vi "Panel Resized.vi"(6 "Sizing Refnums":T2, 8 "error in (no error)":errorcluster, 9 "Origin":cluster{"H":i16, "V":i16}, 10 "NewBnds":T1, 11 "Size Constraints":cluster{"min tab width":i32, "w/h":dbl}) -> (0 "error out":errorcluster)   [LabVIEW 2019]
uses:
  <vilib>/Utility/miscctls.llb/LVRectTypeDef.ctl
  <vilib>/Utility/miscctls.llb/LVRowAndColumnTypeDef.ctl
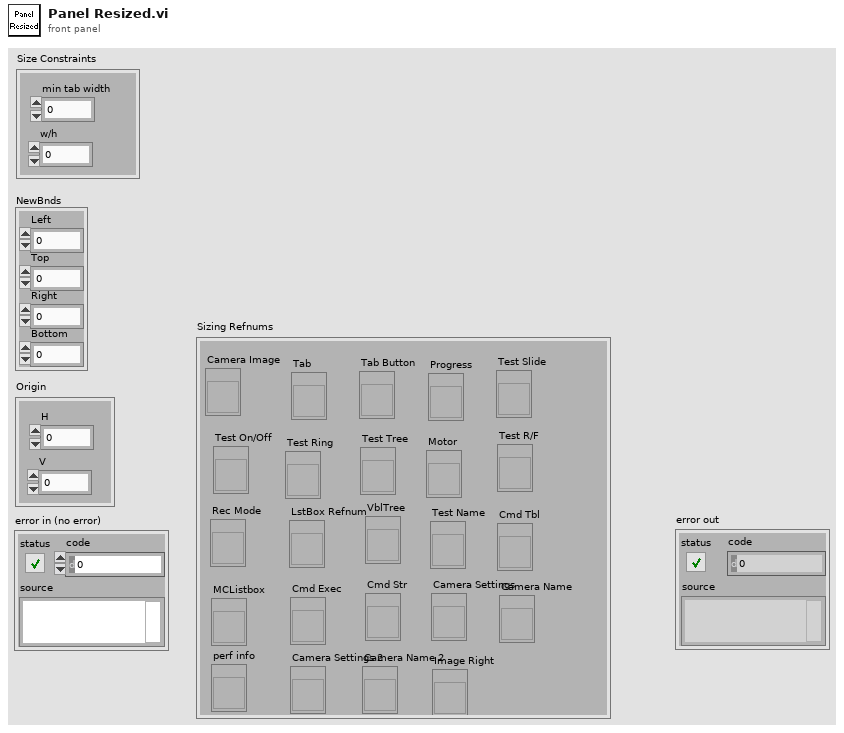
[diagram p1: front panel]
types:
  T1 = typedef "LVRectTypeDef.ctl" = cluster{"Left":i16, "Top":i16, "Right":i16, "Bottom":i16}
  T2 = cluster{"Camera Image":refnum<vi>, "Tab":refnum<vi>, "Tab Button":refnum<vi>, "Rec Mode":refnum<vi>, "Test Slide":refnum<vi>, "Test On/Off":refnum<vi>, "Test Ring":refnum<vi>, "Test R/F":refnum<vi>, "Test Name":refnum<vi>, "Motor":refnum<vi>, "Progress":refnum<vi>, "LstBox Refnum":refnum<vi>, "Test Tree":refnum<vi>, "VblTree":refnum<vi>, "Cmd Tbl":refnum<vi>, "MCListbox":refnum<vi>, "Cmd Exec":refnum<vi>, "Cmd Str":refnum<vi>, "Camera Settings":refnum<vi>, "Camera Name":refnum<vi>, "perf info":refnum<vi>, "Camera Settings 2":refnum<vi>, "Camera Name 2":refnum<vi>, "Image Right":refnum<vi>}
  T3 = typedef "LVRowAndColumnTypeDef.ctl" = cluster{"Row":i32, "Column":i32}
  T4 = typedef "LVPositionTypeDef.ctl" = cluster{"Left":i32, "Top":i32}
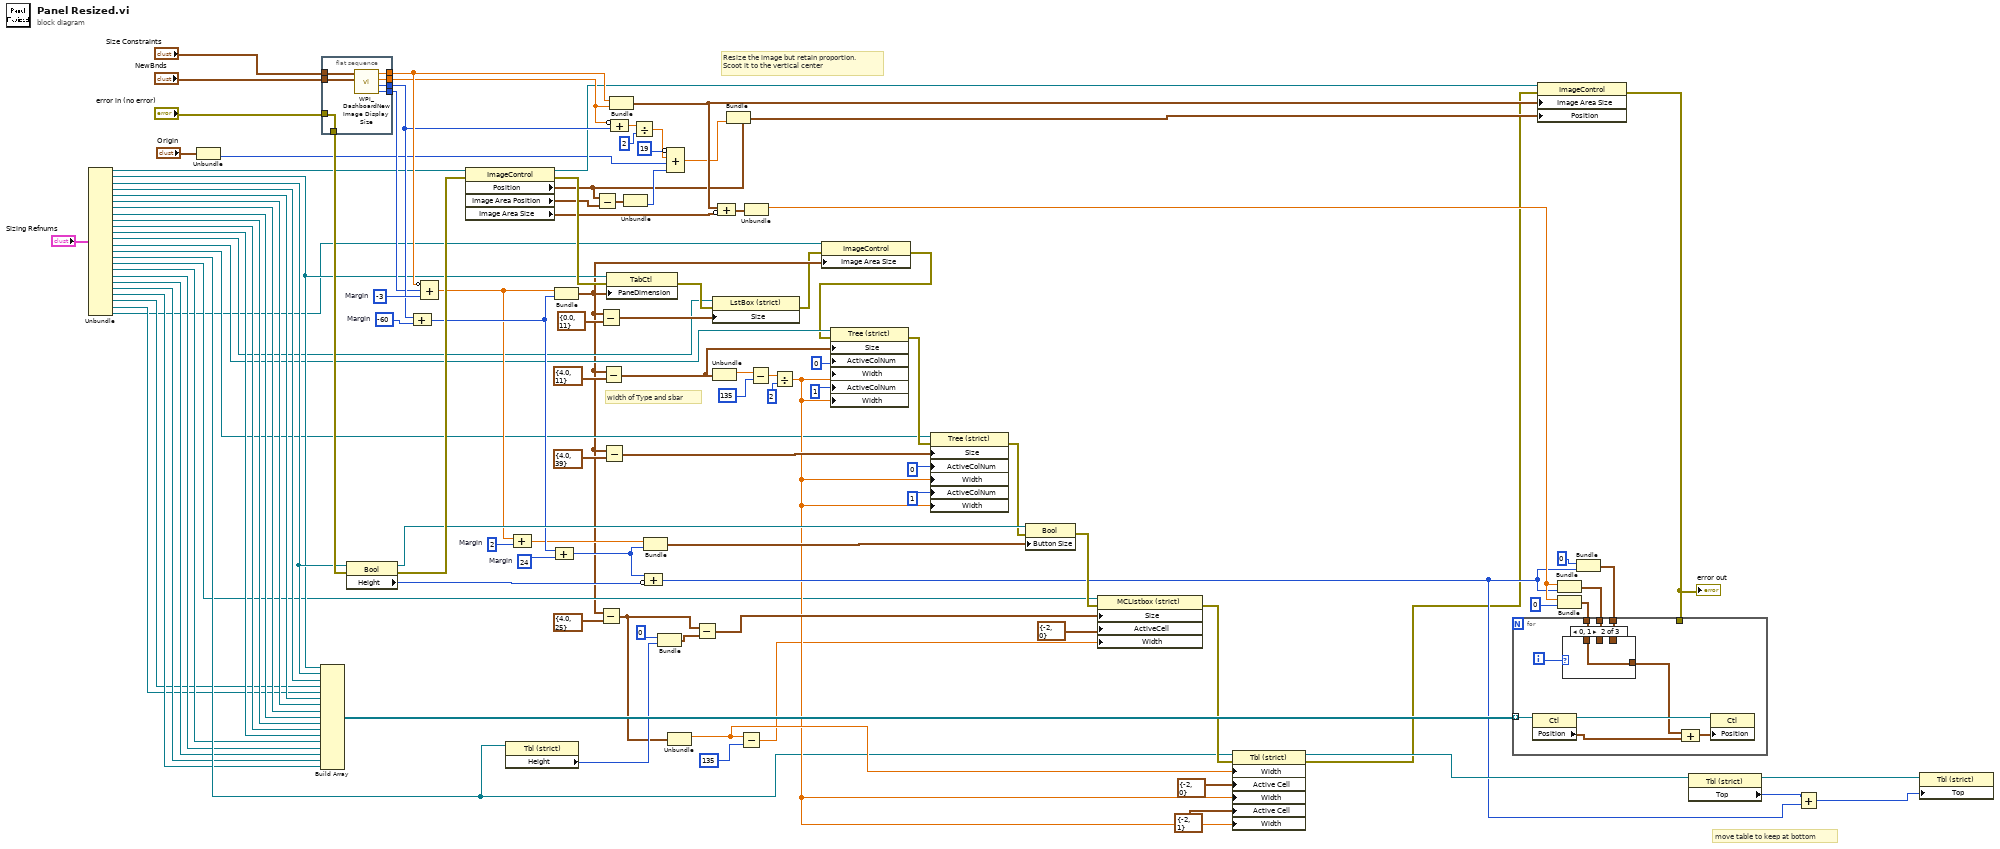
[diagram p0: block diagram]
diagram:
  w98 = 24  # Margin
  w96 = 2  # Margin
  w92 = -60  # Margin
  w102 = -3  # Margin
  # "move table to keep at bottom"
  # "width of Type and sbar"
  # "Resize the image but retain proportion.\nScoot it to the vertical center"
  n1 = Unbundle("Sizing Refnums") -> ("Camera Image"=w66:refnum<vi>, "Tab"=w67:refnum<vi>, "Tab Button"=w75:refnum<vi>, "Rec Mode"=w24:refnum<vi>, "Test Slide"=w23:refnum<vi>, "Test On/Off"=w22:refnum<vi>, "Test Ring"=w21:refnum<vi>, "Test R/F"=w20:refnum<vi>, "Test Name"=w19:refnum<vi>, "Motor"=w18:refnum<vi>, "Progress"=w17:refnum<vi>, "LstBox Refnum"=w16:refnum<vi>, "Test Tree"=w15:refnum<vi>, "VblTree"=w14:refnum<vi>, "Cmd Tbl"=w13:refnum<vi>, "MCListbox"=w12:refnum<vi>, "Cmd Exec"=w11:refnum<vi>, "Cmd Str"=w10:refnum<vi>, "Camera Settings"=w9:refnum<vi>, "Camera Name"=w8:refnum<vi>, "perf info"=w7:refnum<vi>, "Camera Settings 2"=w6:refnum<vi>, "Camera Name 2"=w5:refnum<vi>, "Image Right"=w1:refnum<vi>)
  n2 = Unbundle("Origin") -> ("V"=w72:i16)  [unwired: 1 out]
  n3 = Build Array(w67, w75, w24, w6, w5, w23, w22, w21, w20, w19, w18, w17, w11, w10, w9, w8, w7) -> (w111:refnum<vi>[])
  n4 = flat-sequence {
    tunnel: "NewBnds" -> [w118]
    tunnel: "Size Constraints" -> [w117]
    tunnel: [w116] -> w91
    tunnel: [w115] -> w99
    tunnel: [w114] -> w100
    tunnel: [w113] -> w101
    tunnel: [w112] -> w110
    tunnel: "error in (no error)" -> [w112]
    frame #0 {
      n5 = call <vilib>:"WPI_DashboardNew Image Display Size.vi"("NewBnds"=w118, "Size Constraints"=w117) -> ("Window Width"=w116:i16, "Window Height"=w114:i16, "Height"=w115:dbl, "Width"=w113:dbl)  [unwired: 6 in]
    }
  }
  n6 = property class="Bool"(reference=w75, error in=w110) -> (reference out=w105:refnum<vi>, error out=w109:errorcluster, "Height"=w104:u32)
  n7 = Compound Arithmetic op=unknown(w100, w92) -> (w97:i32)
  n8 = Compound Arithmetic op=ADD(invert w101, w91, w102) -> (w95:dbl)
  n9 = property class="ImageControl"(reference=w66, error in=w109) -> (reference out=w84:refnum<vi>, error out=w108:errorcluster, "Position"=w83:T4, "Image Area Position"=w78:cluster{"Left":i32, "Top":i32}, "Image Area Size"=w89:cluster{"Width":u32, "Height":u32})
  n10 = property class="Tbl (strict)"(reference=w13) -> ("Height"=w42:u32)  [unwired: 1 in, 2 out]
  n11 = Compound Arithmetic op=ADD(w95, w96) -> (w94:dbl)
  n12 = Bundle(w95, w97) -> (w4:cluster{dbl, i32})  [unwired: 1 in]
  n13 = Compound Arithmetic op=ADD(w97, w98) -> (w103:i32)
  n14 = Subtract(x=w83, y=w78) -> (x-y=w85:T4)
  n15 = Subtract(x=w4, y=cluster{dbl, i32} {0.0, 11}) -> (x-y=w64:cluster{dbl, i32})
  n16 = Subtract(x=w4, y=cluster{dbl, i32} {4.0, 25}) -> (x-y=w39:cluster{dbl, i32})
  n17 = Subtract(x=w4, y=cluster{dbl, i32} {4.0, 11}) -> (x-y=w55:cluster{dbl, i32})
  n18 = Subtract(x=w4, y=cluster{dbl, i32} {4.0, 39}) -> (x-y=w60:cluster{dbl, i32})
  n19 = property class="TabCtl"(reference=w67, error in=w108, "PaneDimension"=w4) -> (error out=w65:errorcluster)  [unwired: 1 out]
  n20 = Bundle("Width"=w101, "Height"=w99) -> (w87:cluster{"Width":dbl, "Height":dbl})  [unwired: 1 in]
  n21 = Compound Arithmetic op=ADD(invert w99, w100) -> (w79:dbl)
  n22 = Unbundle(w85) -> ("Top"=w86:i32)  [unwired: 1 out]
  n23 = Divide(x=w79, y=2) -> (x/y=w81:dbl)
  n24 = Bundle(w94, w103) -> (w93:cluster{dbl, i32})  [unwired: 1 in]
  n25 = Compound Arithmetic op=ADD(w103, invert w104) -> (w34:u32)
  n26 = Bundle(0, "Height"=w42) -> (w40:cluster{i32, "Height":u32})  [unwired: 1 in]
  n27 = Compound Arithmetic op=ADD(invert 19, w81, w72, w86) -> (w82:dbl)
  n28 = Unbundle(w39) -> (w29:dbl)  [unwired: 1 out]
  n29 = Subtract(x=w39, y=w40) -> (x-y=w38:cluster{dbl, u32})
  n30 = property class="LstBox (strict)"(reference=w16, error in=w65, "Size"=w64) -> (error out=w3:errorcluster)  [unwired: 1 out]
  n31 = Unbundle(w55) -> (w54:dbl)  [unwired: 1 out]
  n32 = Compound Arithmetic op=ADD(w87, invert w89) -> (w90:cluster{"Width":dbl, "Height":dbl})
  n33 = Bundle(cluster=w83, "Top"=w82) -> (w88:T4)  [unwired: 1 in]
  n34 = Subtract(x=w29, y=135) -> (x-y=w26:dbl)
  n35 = Unbundle(w90) -> ("Width"=w106:dbl)  [unwired: 1 out]
  n36 = Subtract(x=w54, y=135 ("Active Cell:Active Column Number")) -> (x-y=w50:dbl)
  n37 = Divide(x=w50, y=2 ("Active Cell:Active Column Number")) -> (x/y=w27:dbl)
  n38 = property class="ImageControl"(reference=w1, error in=w3, "Image Area Size"=w4) -> (error out=w2:errorcluster)  [unwired: 1 out]
  n39 = property class="Tree (strict)"(reference=w15, error in=w2, "Size"=w55, "ActiveColNum"=0 ("Active Cell:Active Column Number"), "Width"=w27, "ActiveColNum"=1 ("Active Cell:Active Column Number"), "Width"=w27) -> (error out=w59:errorcluster)  [unwired: 1 out]
  n40 = property class="Tree (strict)"(reference=w14, error in=w59, "Size"=w60, "ActiveColNum"=0 ("Active Cell:Active Column Number"), "Width"=w27, "ActiveColNum"=1 ("Active Cell:Active Column Number"), "Width"=w27) -> (error out=w58:errorcluster)  [unwired: 1 out]
  n41 = property class="Bool"(reference=w105, error in=w58, "Button Size"=w93) -> (error out=w46:errorcluster)  [unwired: 1 out]
  n42 = property class="MCListbox (strict)"(reference=w12, error in=w46, "Size"=w38, "ActiveCell"=T3 {"Row"=-2, "Column"=0} ("Active Cell:Active Cell"), "Width"=w26) -> (error out=w43:errorcluster)  [unwired: 1 out]
  n43 = property class="Tbl (strict)"(reference=w13, error in=w43, "Width"=w29, "Active Cell"=T3 {"Row"=-2, "Column"=0} ("Active Cell:Active Cell"), "Width"=w27, "Active Cell"=T3 {"Row"=-2, "Column"=1} ("Active Cell:Active Cell"), "Width"=w27) -> (reference out=w37:refnum<vi>, error out=w32:errorcluster)
  n44 = property class="ImageControl"(reference=w84, error in=w32, "Image Area Size"=w87, "Position"=w88) -> (error out=w71:errorcluster)  [unwired: 1 out]
  "error out" <- w71
  n45 = Bundle("Width"=w106, w34) -> (w77:cluster{"Width":dbl, u32})  [unwired: 1 in]
  n46 = Bundle("Width"=w106, 0) -> (w76:cluster{"Width":dbl, i32})  [unwired: 1 in]
  n47 = Bundle(0, w34) -> (w47:cluster{i32, u32})  [unwired: 1 in]
  n48 = for {
    tunnel: w111 -> [w127] mode=indexing
    tunnel: w77 -> [w121]
    tunnel: w76 -> [w122]
    tunnel: w71 -> [_]
    tunnel: w47 -> [w120]
    i -> [w123]
    n49 = property class="Ctl"(reference=w127) -> (reference out=w126:refnum<vi>, "Position"=w125:T4)  [unwired: 1 in, 1 out]
    n50 = case shown="0, 1" w123 {
      tunnel: w122 -> [_ w129 _]
      tunnel: w121 -> [_ _ w130]
      tunnel: w120 -> [w128 _ _]
      tunnel: [w128 w129 w130] -> w119
      frame Default {
      }
      frame 0, 1 {
      }
      frame 2..4 {
      }
    }
    n51 = Compound Arithmetic op=ADD(w119, w125) -> (w124:cluster{dbl, u32})
    n52 = property class="Ctl"(reference=w126, "Position"=w124) -> ()  [unwired: 1 in, 2 out]
  }
  n53 = property class="Tbl (strict)"(reference=w37) -> (reference out=w36:refnum<vi>, "Top"=w35:i32)  [unwired: 1 in, 1 out]
  n54 = Add(x=w35, y=w34) -> (x+y=w33:u32)
  n55 = property class="Tbl (strict)"(reference=w36, "Top"=w33) -> ()  [unwired: 1 in, 2 out]
